vi "Read database.vi"(5 "String":string) -> (0 "error out":errorcluster, 1 "Operator Id":string[](array[string]), 2 "DB Data":T1)   [LabVIEW 2015]
uses:
  <vilib>/addons/database/Connection.llb/DB Tools Open Connec (String).vi
  Galobal variable_TI.vi
  <vilib>/addons/database/_DB Variant To Data/Database Variant To Data.xnode
  <vilib>/addons/database/NI_Database_API.lvlib
panel:
  out "appended array 4":string[](array[string])
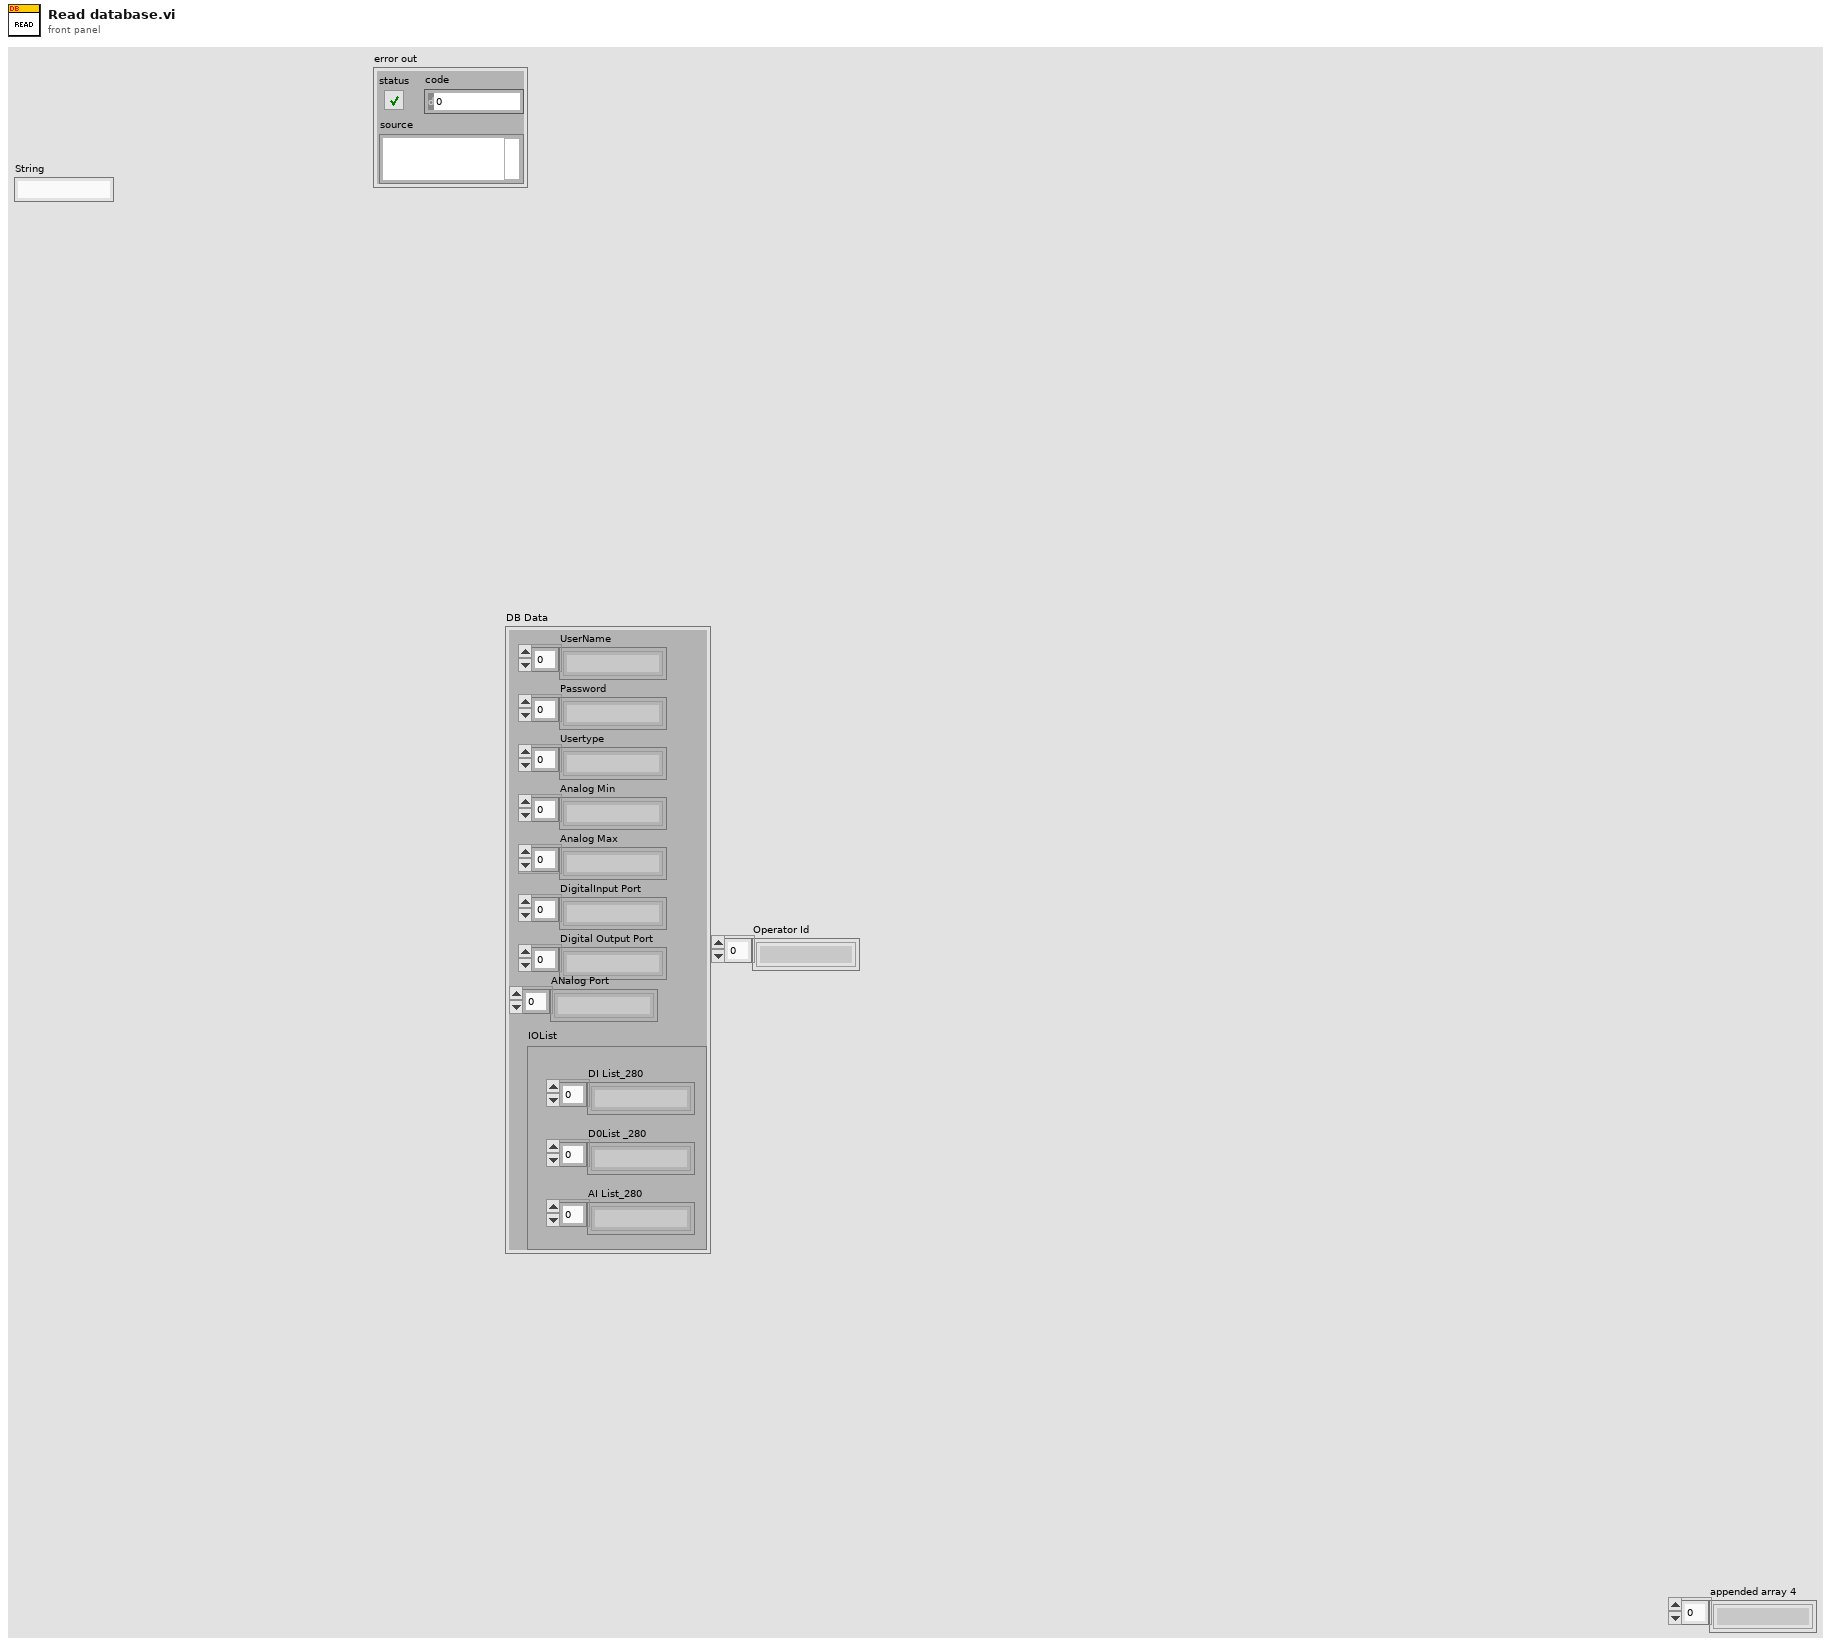
[diagram p1: front panel]
types:
  T1 = cluster{"UserName":string[], "Password":string[], "Usertype":string[], "Analog Min":string[], "Analog Max":string[], "DigitalInput Port":string[], "Digital Output Port":string[], "ANalog Port":string[], "IOList":cluster{"DI List_280":string[], "D0List _280":string[], "AI List_280":string[]}}
  T2 = cluster{"IL Sensor1_Max AI0":dbl, "IL Sensor1_Min AI0":dbl, "IL Sensor1_Max AI1":dbl, "IL Sensor1_ Min AI1":dbl, "IL Sensor_Max (AI9)":dbl, "IL Sensor_Min  (AI9)":dbl, "IL Sensor_Max (AI10)":dbl, "IL Sensor_Min(AI10)":dbl, "IL Sensor_Max (AI11)":dbl, "IL Sensor_Min (AI11)":dbl, "IL Sensor_Max (AI12)":dbl, "IL Sensor_Min (AI12":dbl}
  T3 = cluster{"To-A":timestamp, "From-A":timestamp, "From-B":timestamp, "To-B":timestamp, "From-C 1":timestamp, "To-C 1":timestamp, "From-C 2":timestamp, "To-C 2":timestamp, "Shift":string}[]
  T4 = typedef "NI_Database_API.lvlib/Conn ObjectReference.ctl" = refnum<k1>
  T5 = cluster{"DI List_280":string[], "D0List _280":string[], "AI List_280":string[]}
  T6 = cluster{"To-A":timestamp, "From-A":timestamp, "From-B":timestamp, "To-B":timestamp, "From-C 1":timestamp, "To-C 1":timestamp, "From-C 2":timestamp, "To-C 2":timestamp, "Shift":string}
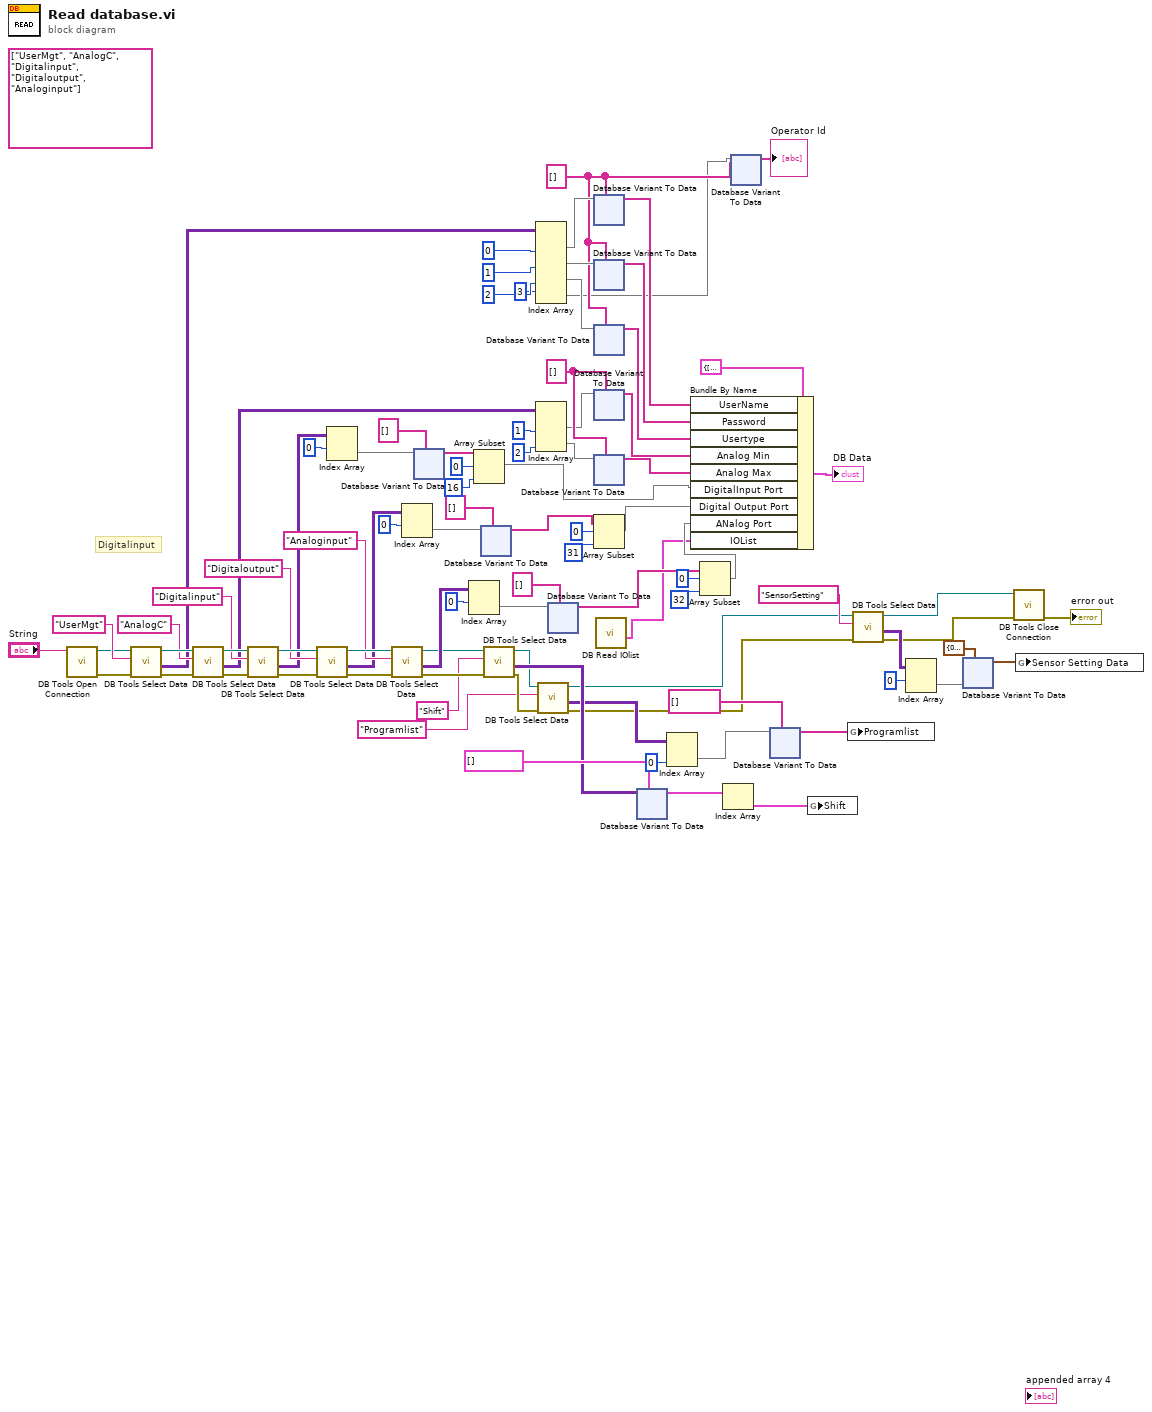
[diagram p0: block diagram]
diagram:
  w82 = string[] []
  (unwired) string[] ["UserMgt", "AnalogC", "Digitalinput", "Digitaloutput", "Analoginput"]
  w4 = string[] []
  # "Digitalinput"
  n1 = call-poly <vilib>:"DB Tools Open Connection.vi"("connection information"="String") -> ("error out"=w50:errorcluster, "connection reference"=w51:T4)  [unwired: 7 in]
  n2 = call <vilib>:"DB Tools Select Data.vi"("error in (no error)"=w50, "table"="UserMgt", "connection reference"=w51) -> ("error out"=w64:errorcluster, "data"=w49:variant[][], "connection reference out"=w62:T4)  [unwired: 3 in]
  n3 = call <vilib>:"DB Tools Select Data.vi"("error in (no error)"=w64, "table"="AnalogC", "connection reference"=w62) -> ("error out"=w63:errorcluster, "data"=w48:variant[][], "connection reference out"=w61:T4)  [unwired: 3 in]
  n4 = call <vilib>:"DB Tools Select Data.vi"("error in (no error)"=w63, "table"="Digitalinput", "connection reference"=w61) -> ("error out"=w57:errorcluster, "data"=w47:variant[][], "connection reference out"=w56:T4)  [unwired: 3 in]
  n5 = call <vilib>:"DB Tools Select Data.vi"("error in (no error)"=w57, "table"="Digitaloutput", "connection reference"=w56) -> ("error out"=w53:errorcluster, "data"=w46:variant[][], "connection reference out"=w54:T4)  [unwired: 3 in]
  n6 = Index Array(array=w47, index (row)=0 ("disabled index (col)")) -> (element=w84:variant[])  [unwired: 1 in]
  n7 = call <vilib>:"DB Tools Select Data.vi"("error in (no error)"=w53, "table"="Analoginput", "connection reference"=w54) -> ("error out"=w40:errorcluster, "data"=w45:variant[][], "connection reference out"=w39:T4)  [unwired: 3 in]
  n8 = Index Array(array=w46, index (row)=0 ("disabled index (col)")) -> (element=w85:variant[])  [unwired: 1 in]
  n9 = xnode "Database Variant To Data"("database variant"=w84, "type"=string[] []) -> ("data"=w36:string[])  [unwired: 1 in, 1 out]
  n10 = Index Array(array=w45, index (row)=0 ("disabled index (col)")) -> (element=w88:variant[])  [unwired: 1 in]
  n11 = Array Subset(array=w36, index=0, length=16) -> (w33:string[])
  n12 = xnode "Database Variant To Data"("database variant"=w85, "type"=string[] []) -> ("data"=w31:string[])  [unwired: 1 in, 1 out]
  n13 = call <vilib>:"DB Tools Select Data.vi"("error in (no error)"=w40, "table"="Shift", "connection reference"=w39) -> ("error out"=w22:errorcluster, "data"=w37:variant[][], "connection reference out"=w23:T4)  [unwired: 3 in]
  n14 = Index Array(array=w49, index (col) #1=0 ("disabled index (col)"), index (col) #2=1 ("index (col)"), index (col) #3=2 ("index (col)"), index (row) #4=3 ("disabled index (row)")) -> (element #1=w75:variant[], element #2=w72:variant[], element #3=w71:variant[], element #4=w2:variant[])  [unwired: 4 in]
  n15 = Index Array(array=w48, index (col) #1=1 ("disabled index (col)"), index (col) #2=2 ("index (col)")) -> (element #1=w80:variant[], element #2=w81:variant[])  [unwired: 2 in]
  n16 = call <vilib>:"DB Tools Select Data.vi"("error in (no error)"=w22, "table"="Programlist", "connection reference"=w23) -> ("error out"=w8:errorcluster, "data"=w20:variant[][], "connection reference out"=w9:T4)  [unwired: 3 in]
  n17 = xnode "Database Variant To Data"("database variant"=w88, "type"=string[] []) -> ("data"=w26:string[])  [unwired: 1 in, 1 out]
  n18 = xnode "Database Variant To Data"("database variant"=w75, "type"=w4) -> ("data"=w70:string[])  [unwired: 1 in, 1 out]
  n19 = xnode "Database Variant To Data"("database variant"=w72, "type"=w4) -> ("data"=w69:string[])  [unwired: 1 in, 1 out]
  n20 = xnode "Database Variant To Data"("database variant"=w71, "type"=w4) -> ("data"=w68:string[])  [unwired: 1 in, 1 out]
  n21 = xnode "Database Variant To Data"("database variant"=w80, "type"=w82) -> ("data"=w67:string[])  [unwired: 1 in, 1 out]
  n22 = xnode "Database Variant To Data"("database variant"=w81, "type"=w82) -> ("data"=w66:string[])  [unwired: 1 in, 1 out]
  n23 = Array Subset(array=w31, index=0, length=31) -> (w29:string[])
  n24 = call "DB Read IOlist.vi"() -> ("output cluster"=w24:T5)  [unwired: 11 in]
  n25 = xnode "Database Variant To Data"("database variant"=w37, "type"=T3 []) -> ("data"=w41:T3)  [unwired: 1 in, 1 out]
  n26 = Index Array(array=w20, index (col)=0 ("disabled index (col)")) -> (element=w19:variant[])  [unwired: 1 in]
  n27 = Array Subset(array=w26, index=0, length=32) -> (w25:string[])
  n28 = Bundle By Name(cluster=T1 {"UserName"=[], "Password"=[], "Usertype"=[], "Analog Min"=[], "Analog Max"=[], "DigitalInput Port"=[], "Digital Output Port"=[], "ANalog Port"=[], "IOList"={"DI List_280"=[" Start PB (P0.0) ", "Emergency Stop (P0.1)", "Reset PB (P0.2)", "Home PB (P0.3)", "Main Pressure Signal (P0.4)", "Safety Signal-1 (P0.5)", "Safety Signal-2 (P0.6)", "Fixture Sliding Servo Home RS (P0.7)", "Fixture Sliding Servo Fault Signal (P0.8)", "LCD pressing Servo Home RS (P0.9)", "LCD pressing Servo fault Signal (P0.10)", "Spare", "Spare", "Spare", "Spare", "Model conformation PX-1 (AI2)", "Model conformation PX-2 (AI3)", "Diffuser height checking Sensor-1 (AI4)", "Diffuser height checking Sensor-2 (AI5)", "Panel Door Open Signal (AI6)", "Component CNF Sensor on Ionizer (AI7)", "Bi-adhesive tube Waste Collection bin CNF Sensor (AI8)", "Photo Prism presence Sensor (AI9)", "Lightbox presence CNF Sensor (AI10)", "Diffuser presence CNF Sensor (AI11)", "Photo prism height checking UP CYL Rs (AI12)", "Photo prism height checking DWN CYL  Rs (AI13)", "Camera slide Cyl Fwd Rs (AI14)", "Camera slide Cyl Rev Rs (AI15)", "LCD Display Rotating Unit Actuator Cyl CW PX (AI16)", "LCD Display Rotating Unit Actuator Cyl CCW PX (AI17)", "Fixture clamping Cyl Fwd Rs (AI18)", "Fixture clamping Cyl Rev Rs (AI19)", "Clip pulling unit Cyl Fwd Rs (AI20)", "Clip pulling unit Cyl Rev Rs (AI21)", "Clip clamp unit Cyl Fwd Rs (A22)", "Clip clamp unit Cyl Rev Rs (AI23)", "Barcode Scanner Ready Signal (AI24)", "Spare", "Spare", "Spare", "Spare", "Spare", "Spare", "Spare"], "D0List _280"=["Ionizer ON Sol (P0.16)", "Fixture Slide Servo Fault Reset (P0.17)", "LCD pressing servo Fault Reset (P0.18)", "Fixture Slide servo Brake ON Cmd (P0.19)", "Fixture Slide Servo Direction Command (P0.20)", "LCD pressing Servo Direction Command (P0.21)", "LCD pressing Servo Brake ON Cmd (P0.22)", "Photo prism height checking UP CYL Sol (P0.23)", "Photo prism height checking DWN CYL  Sol (P0.24)", "Camera slide Cyl Fwd Sol (P0.25)", "Camera slide Cyl Rev Sol (P0.26)", "LCD Display Rotating Unit Actuator Cyl CW Sol (P0.27)", "LCD Display Rotating Unit Actuator Cyl CCW Sol (P0.28)", "Fixture clamping Cyl Fwd Sol (P0.29)", "Fixture clamping Cyl Rev Sol (P0.30)", "Clip pulling unit Cyl Fwd Sol (P0.31)", "Clip pulling unit Cyl Rev Sol (P1.0)", "Clip clamp unit Cyl Up Sol (P1.1)", "Clip clamp unit Cyl Dwn Sol (P1.2)", "Optional required based Barcode Trigger Cmd (P1.3)", "TWL Red /Fault with Buzzer (P1.4)", "TWL Green/OK (P1.5)", "TWL Yellow/ Running (P1.6)", "Spare", "Spare", "Spare", "Spare", "Spare", "Fixture Slide Servo Pulse Command (P2.4)", "LCD pressing Servo Pulse Command (P2.5)", "Spare", "Spare"], "AI List_280"=["Loadcell Signal For LCD PRESSING (AI0)", "LVDT SIGNAL FOR PHOTO PRISM HEIGHT CHECK (AI1)"]}} ("DB Data 2"), "UserName"=w70, "Password"=w69, "Usertype"=w68, "Analog Min"=w67, "Analog Max"=w66, "DigitalInput Port"=w33, "Digital Output Port"=w29, "ANalog Port"=w25, "IOList"=w24) -> (→"DB Data":T1)
  n29 = Index Array(array=w41) -> (element=w5:T6)  [unwired: 1 in]
  n30 = xnode "Database Variant To Data"("database variant"=w2, "type"=w4) -> ("data"=→"Operator Id":string[])  [unwired: 1 in, 1 out]
  n31 = xnode "Database Variant To Data"("database variant"=w19, "type"=string[] []) -> ("data"=w17:string[])  [unwired: 1 in, 1 out]
  n32 = global write "Galobal variable_TI.vi" "Shift"(w5) -> ()
  n33 = global write "Galobal variable_TI.vi" "Programlist"(w17) -> ()
  n34 = call <vilib>:"DB Tools Select Data.vi"("error in (no error)"=w8, "table"="SensorSetting", "connection reference"=w9) -> ("error out"=w6:errorcluster, "data"=w12:variant[][], "connection reference out"=w7:T4)  [unwired: 3 in]
  n35 = Index Array(array=w12, index (row)=0) -> (element=w14:variant[])  [unwired: 1 in]
  n36 = xnode "Database Variant To Data"("database variant"=w14, "type"=T2 {"IL Sensor1_Max AI0"=0.0, "IL Sensor1_Min AI0"=0.0, "IL Sensor1_Max AI1"=0.0, "IL Sensor1_ Min AI1"=0.0, "IL Sensor_Max (AI9)"=0.0, "IL Sensor_Min  (AI9)"=0.0, "IL Sensor_Max (AI10)"=0.0, "IL Sensor_Min(AI10)"=0.0, "IL Sensor_Max (AI11)"=0.0, "IL Sensor_Min (AI11)"=0.0, "IL Sensor_Max (AI12)"=0.0, "IL Sensor_Min (AI12"=0.0} ("Sensor Setting Data")) -> ("data"=w10:T2)  [unwired: 1 in, 1 out]
  n37 = call <vilib>:"DB Tools Close Connection.vi"("error in (no error)"=w6, "connection reference"=w7) -> ("error out"=→"error out":errorcluster)  [unwired: 5 in]
  n38 = global write "Galobal variable_TI.vi" "Sensor Setting Data"(w10) -> ()
